vi "USB_Communication_Polar.vi"(7 "Polarity":enum16{"POS ", "NEG "}(ring), 8 "error in (no error)":errorcluster, 9 "number":i32, 10 "string":string, 11 "APS PORT":refnum<visa-resource-name>) -> (0 "error out":errorcluster, 2 "read buffer":string, 3 "APS PORT Out":refnum<visa-resource-name>)   [LabVIEW 2025]
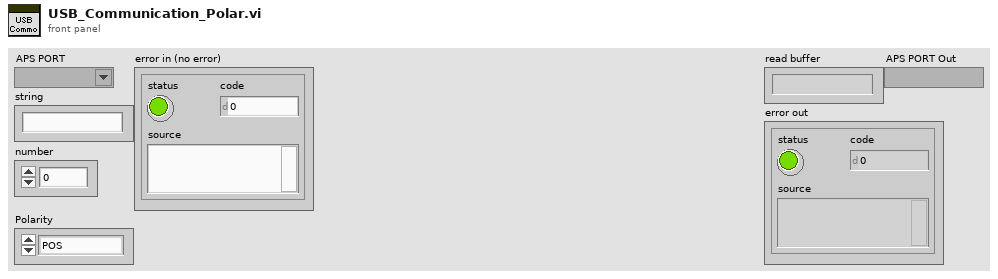
[diagram p1: front panel]
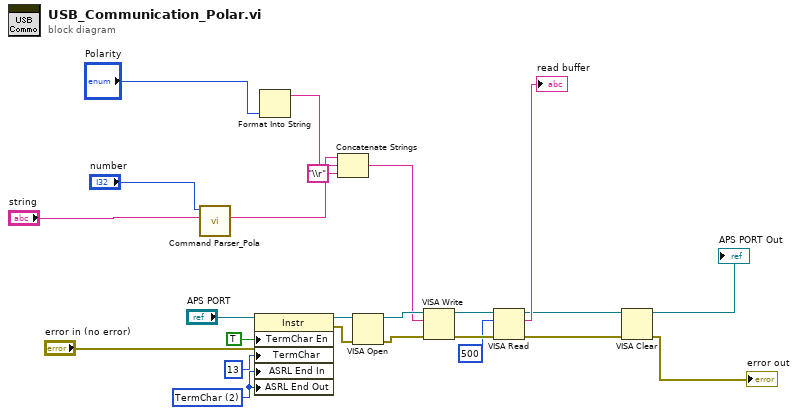
[diagram p0: block diagram]
diagram:
  w19 = u16 2 items=["None", "Last Bit", "TermChar", "Break"] ("Serial Settings:End Mode for Writes")
  n1 = call "Command Parser_Pola.vi"("Task IN"="string", "Numeric"="number") -> ("Task Out"=w3:string)  [unwired: 9 in]
  n2 = property class="Instr"(reference="APS PORT", error in="error in (no error)", "TermChar En"=TRUE ("Message Based Settings:Termination Character Enable"), "TermChar"=u8 13 ("Message Based Settings:Termination Character"), "ASRL End In"=w19, "ASRL End Out"=w19) -> (reference out=w24:refnum<visa-resource-name>, error out=w23:errorcluster)
  n3 = Format Into String("Polarity") -> (resulting string=w2:string)  [unwired: 3 in, 1 out]
  n4 = Concatenate Strings(w3, w2, "\\r" ("string")) -> (w4:string)
  n5 = VISA Open(error in (no error)=w23, VISA resource name=w24) -> (VISA resource name=w16:refnum<visa-resource-name>, error out=w15:errorcluster)  [unwired: 3 in]
  n6 = VISA Write(VISA resource name=w16, write buffer=w4, error in (no error)=w15) -> (VISA resource name out=w13:refnum<visa-resource-name>, error out=w14:errorcluster)  [unwired: 1 out]
  n7 = VISA Read(VISA resource name=w13, byte count=u32 500, error in (no error)=w14) -> (VISA resource name out=w11:refnum<visa-resource-name>, read buffer=→"read buffer":string, error out=w10:errorcluster)  [unwired: 1 out]
  n8 = VISA Clear(VISA resource name=w11, error in (no error)=w10) -> (VISA resource name out=→"APS PORT Out":refnum<visa-resource-name>, error out=→"error out":errorcluster)
